vi "movie_data_file_path_choose2.vi"(1 "CM":i32) -> (0 "appended path":path)   [LabVIEW 2014]
panel:
  out "name":string
  out "path":path
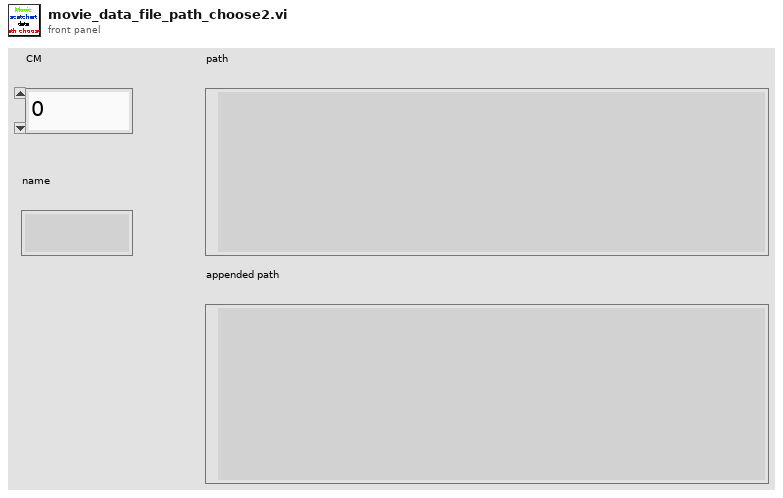
[diagram p1: front panel]
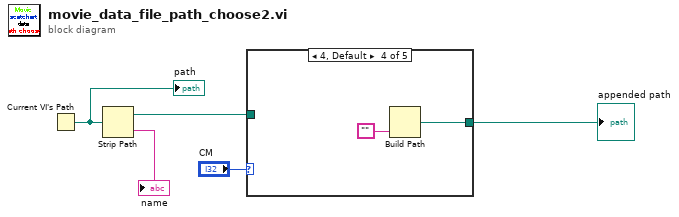
[diagram p0: block diagram]
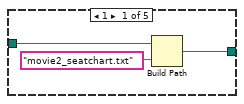
[diagram p2: hidden frame]
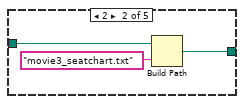
[diagram p3: hidden frame]
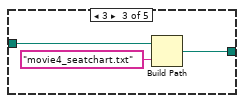
[diagram p4: hidden frame]
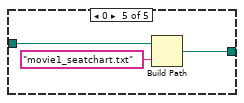
[diagram p5: hidden frame]
diagram:
  n1 = Current VI's Path() -> (path=w5:path)
  "path" <- w5
  n2 = Strip Path(path=w5) -> (stripped path=w4:path, name=→"name":string)
  n3 = case shown="4, Default" "CM" {
    tunnel: w4 -> [w8 w11 w14 _ w19]
    tunnel: [w6 w9 w12 w16 w17] -> w3
    frame 1 {
      n4 = Build Path(base path=w8, name or relative path="movie2_seatchart.txt") -> (appended path=w6:path)
    }
    frame 2 {
      n5 = Build Path(base path=w11, name or relative path="movie3_seatchart.txt") -> (appended path=w9:path)
    }
    frame 3 {
      n6 = Build Path(base path=w14, name or relative path="movie4_seatchart.txt") -> (appended path=w12:path)
    }
    frame 4, Default {
      n7 = Build Path(name or relative path="") -> (appended path=w16:path)  [unwired: 1 in]
    }
    frame 0 {
      n8 = Build Path(base path=w19, name or relative path="movie1_seatchart.txt") -> (appended path=w17:path)
    }
  }
  "appended path" <- w3
